vi "ChipKit RGB LED.vi"() -> ()   [LabVIEW 2011, in "LabVIEW Interface for ChipKit.lvlib"]
doc: "An example that uses I2C to control a BlinkM."
uses:
  vi.lib/LabVIEW Interface for ChipKit/LabVIEW Interface for ChipKit.lvlib
  vi.lib/LabVIEW Interface for ChipKit/Private/Type Defs/Chipkit Configuration.ctl
  vi.lib/LabVIEW Interface for ChipKit/Private/Type Defs/Board Type.ctl
  vi.lib/LabVIEW Interface for ChipKit/Private/Type Defs/RGB LED Pins.ctl
  vi.lib/LabVIEW Interface for ChipKit/Private/Type Defs/PWM Pin.ctl
panel:
  in  "RGB LED Pins":T1
  in  "Stop Button":bool
  out "LED Color":u32(colorbox)
  in  "Blue":u8(slide) scale=0.0..255.0
  in  "Green":u8(slide) scale=0.0..255.0
  in  "Red":u8(slide) scale=0.0..255.0
  in  "ChipKit Configuration":T3={"COM Port"="COM3", "Board Type"=enum."ChipKit uC32"}
  # "Color Settings"
  # "chipKIT Settings"
  # "RGB LED Settings"
  # "RGB LED Example\n\nThis example demonstrates how control an RGB LEDLabVIEW and a ChipKit microcontroller.\n\nInstructions\n1. Select the COM Port associated with the ChipKit.\n2. Select the Board Type.\n3. Select the PWM pins connected to the Red, Green, and Blue LED Pins.\n3. Click the Run Arrow.\n5. Adjust the Color Sliders (Red, Green and Blue) to change the RGB LED's output color."
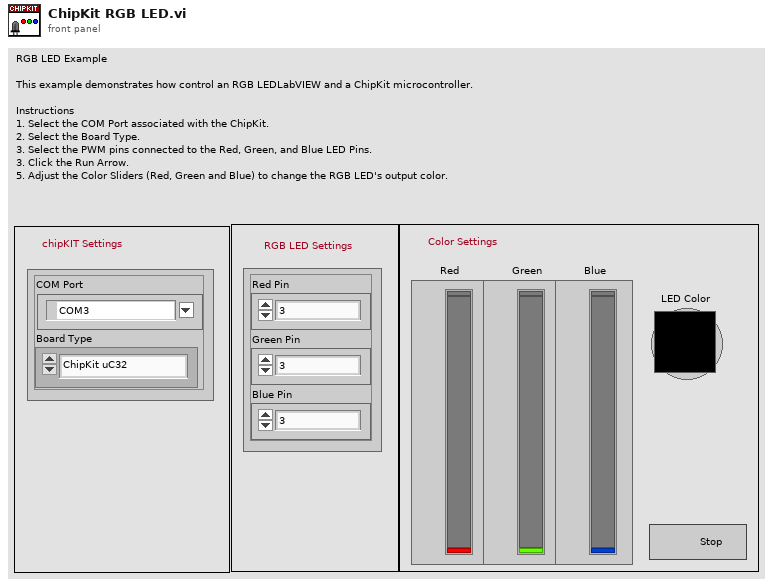
[diagram p1: front panel]
types:
  T1 = typedef "LabVIEW Interface for ChipKit.lvlib/RGB LED Pins.ctl" = cluster{"Red Pin ":T2, "Green Pin":T2, "Blue Pin":T2}
  T2 = typedef "LabVIEW Interface for ChipKit.lvlib/PWM Pin.ctl" = enum8{"3", "5", "6", "9", "10"}
  T3 = typedef "LabVIEW Interface for ChipKit.lvlib/Chipkit Configuration.ctl" = cluster{"COM Port":refnum<visa-resource-name>, "Board Type":T4}
  T4 = typedef "LabVIEW Interface for ChipKit.lvlib/Board Type.ctl" = enum16{"ChipKit uC32", "ChipKit Uno32", "ChipKit Max32"}
  T5 = typedef "LabVIEW Interface for ChipKit.lvlib/Chipkit Resource.ctl" = cluster{"COM Port":refnum<visa-resource-name>, "Board Type":T4, "Connection Type":T6, "Baud Rate (115200)":u32, "Bytes Per Packet (15)":u32, "DI Port Num Pins":i32, "DO Port Num Pins":i32}
  T6 = typedef "LabVIEW Interface for ChipKit.lvlib/Connection Type.ctl" = enum8{"USB / Serial", "XBEE", "BlueSmirf (Bluetooth)"}
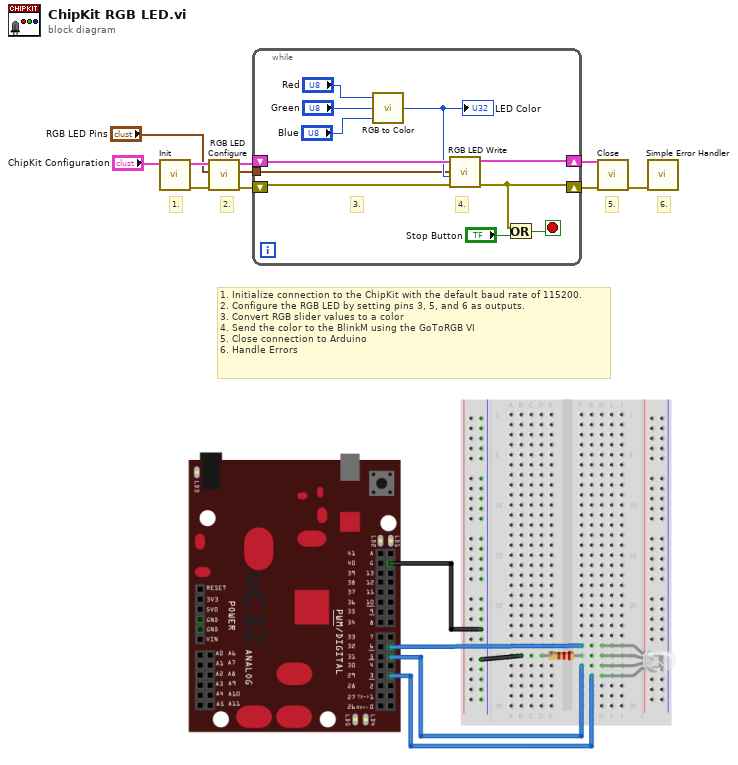
[diagram p0: block diagram]
diagram:
  # "6."
  # "5."
  # "2."
  # "1."
  # "1. Initialize connection to the ChipKit with the default baud rate of 115200.\n2. Configure the RGB LED by setting pins 3, 5, and 6 as outputs.\n3. Convert RGB slider values to a color\n4. Send the color to the BlinkM using the GoToRGB VI\n5. Close connection to Arduino\n6. Handle Errors"
  n1 = call "Init.vi"("ChipKit Configuration"="ChipKit Configuration") -> ("Error Out"=w8:errorcluster, "ChipKit Configuration"=w9:T5)  [unwired: 9 in]
  n2 = call "RGB LED Configure.vi"("Error In"=w8, "RGB LED Pins"="RGB LED Pins", "ChipKit Resource"=w9) -> ("Error Out"=w6:errorcluster, "RGB LED Pins"=w2:T1, "ChipKit Resource"=w7:T5)  [unwired: 6 in]
  n3 = while {
    shift-right: [w21] -> w5
    shift-left: w7 -> [w19]
    shift-right: [w14] -> w4
    shift-left: w6 -> [w20]
    tunnel: w2 -> [w11]
    stop <- w12 stop-if-true
    # "3."
    # "4."
    n4 = call <vilib>:"RGB to Color.vi"("B"="Blue", "G"="Green", "R"="Red") -> ("Color"=w15:u32)
    "LED Color" <- w15
    n5 = call "RGB LED Write.vi"("Error In"=w20, "Color"=w15, "RGB LED Pins"=w11, "ChipKit Resource"=w19) -> ("Error Out"=w14:errorcluster, "ChipKit Resource"=w21:T5)  [unwired: 5 in, 1 out]
    n6 = Or(x=w14, y="Stop Button") -> (x .or. y?=w12:bool)
  }
  n7 = call "Close.vi"("Error In"=w4, "ChipKit Configuration"=w5) -> ("Error Out"=w10:errorcluster)  [unwired: 9 in]
  n8 = call <vilib>:"Simple Error Handler.vi"("error in (no error)"=w10) -> ()  [unwired: 4 in, 5 out]
